vi "Main.vi"() -> ()   [LabVIEW 2020]
doc: "Ce VI modèle est conçu pour le modèle de conception Gestionnaire de messages dans une file d'attente.\n\nLa boucle de gestion d'événements génère des messages en fonction des actions sur l'interface utilisateur.\n\nLa boucle de gestion de messages traite les messages générés par la boucle de gestion d'événements ou par d'autres messages. Les messages sont des valeurs chaîne ; il est donc facile d'ajouter de nouveaux messages à la structure condition Conditions de messages de la boucle de gestion de messages Chaque cluster Message peut en outre fournir une valeur optionnelle pour Données de message, un variant qui peut être converti aux données requises pour un message spécifique."
uses:
  controls/Ctrl_RefPad.ctl
  controls/UI Data.ctl
  support/Message Queue/Enqueue Message (Single).vi
  <vilib>/Utility/error.llb/Error Cluster From Error Code.vi
  <vilib>/ErrorRing/Error Ring.xnode
  support/Message Queue/Message Queue.lvlib
  support/User Event - Stop/User Event - Stop.lvlib
panel:
  in  "Btn_Error_etat":bool caption="Error state"
  in  "Btn_Error":bool caption="Error"
  out "sortie d'erreur":errorcluster
  out "Display":cluster{"Num":dbl, "Char":string}
  in  "Pad":T1
  in  "Btn_Stop":bool
  # "Calculatrice"
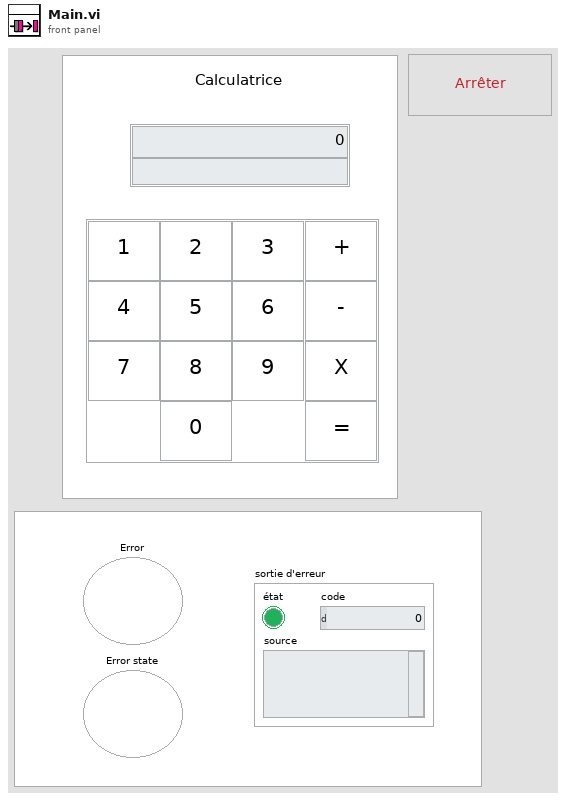
[diagram p1: front panel]
types:
  T1 = cluster{"Btn_1":bool, "Btn_2":bool, "Btn_3":bool, "Btn_4":bool, "Btn_5":bool, "Btn_6":bool, "Btn_7":bool, "Btn_8":bool, "Btn_9":bool, "Btn_0":bool, "Btn_+":bool, "Btn_-":bool, "Btn_X":bool, "Btn_=":bool}
  T2 = cluster{"état":bool, "code":i32, "source":string}
  T3 = typedef "Message Queue.lvlib/All Message Queues.ctl" = cluster{"IU":refnum<queue>}
  T4 = typedef "UI Data.ctl" = cluster{"Event":cluster{"Stop":refnum<user-event>}, "Data":cluster{"Display":cluster{"Num":dbl, "Char":string}, "memory":string}}
  T5 = typedef "Ctrl_RefPad.ctl" = cluster{"BTN_Ref":refnum<vi>, "CharPad":string}
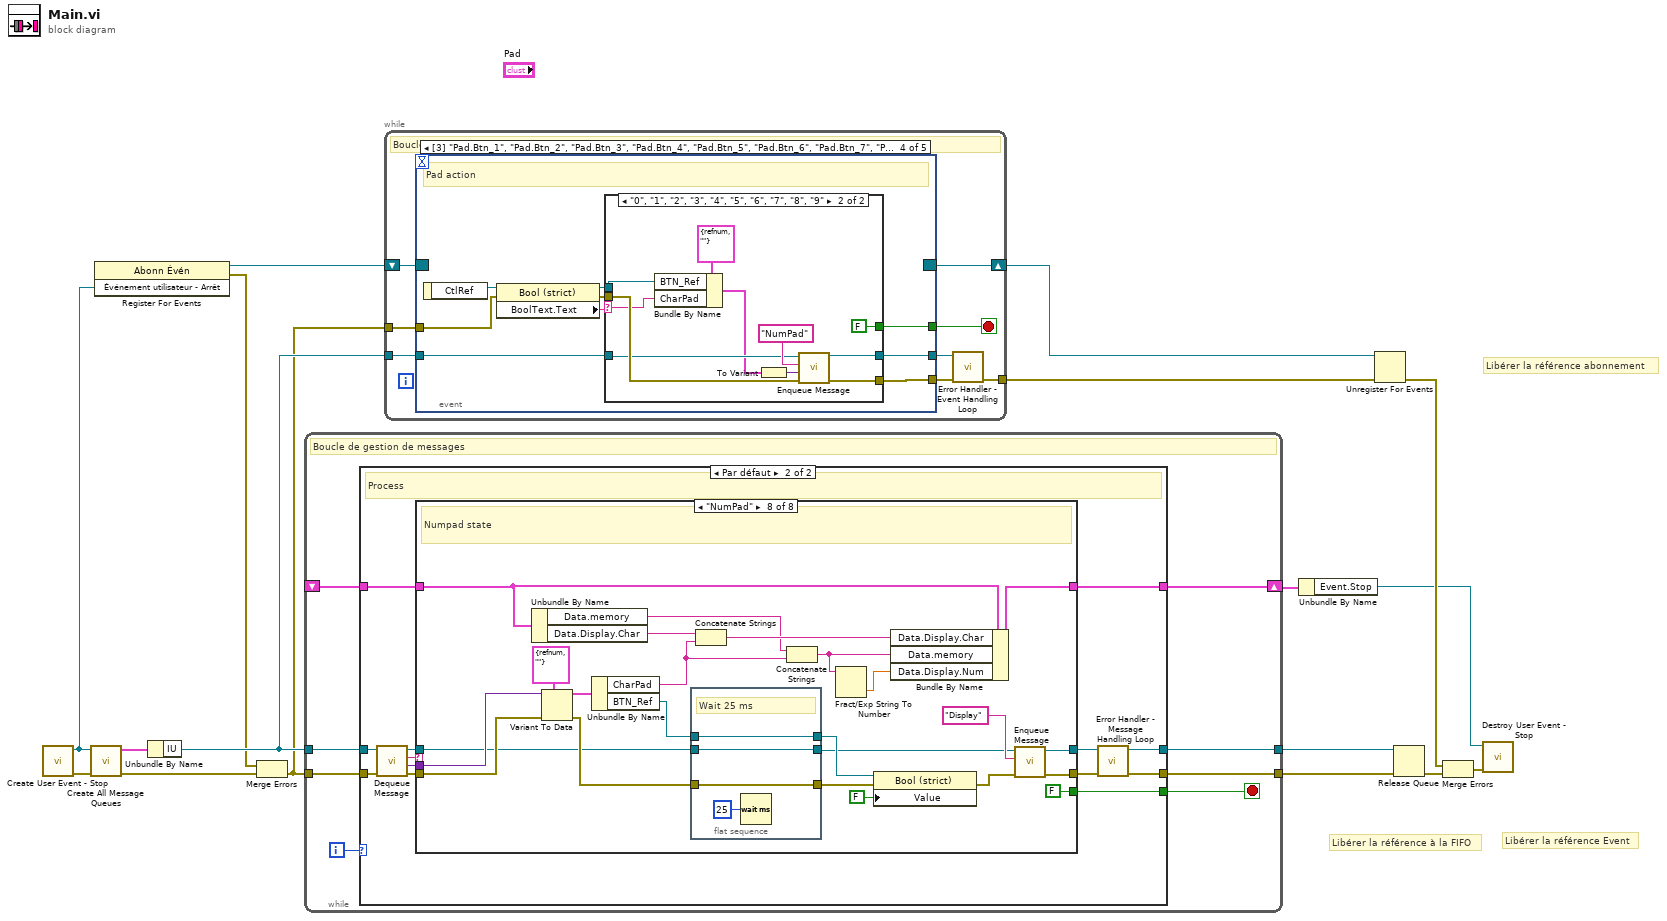
[diagram p0: block diagram]
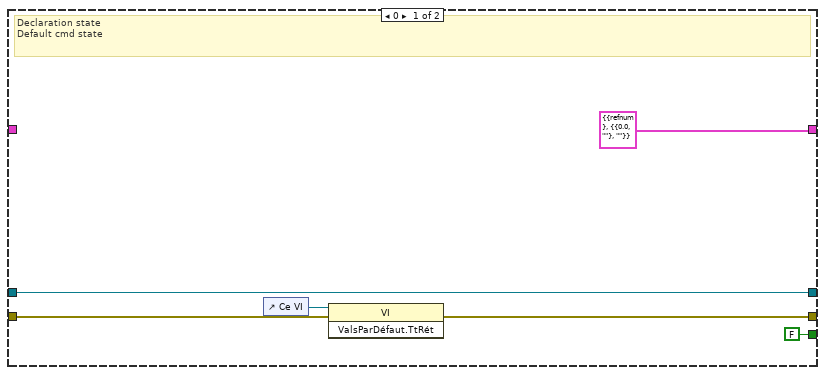
[diagram p2: hidden frame]
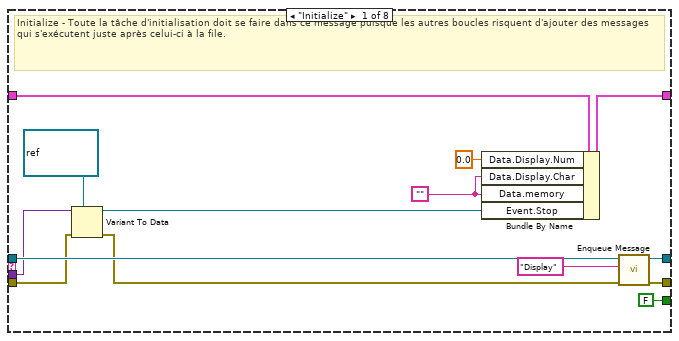
[diagram p3: hidden frame]
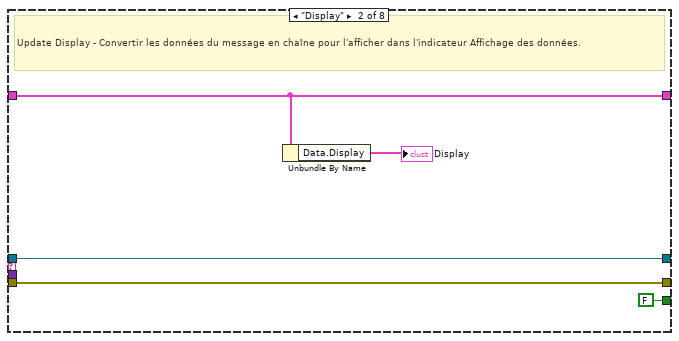
[diagram p4: hidden frame]
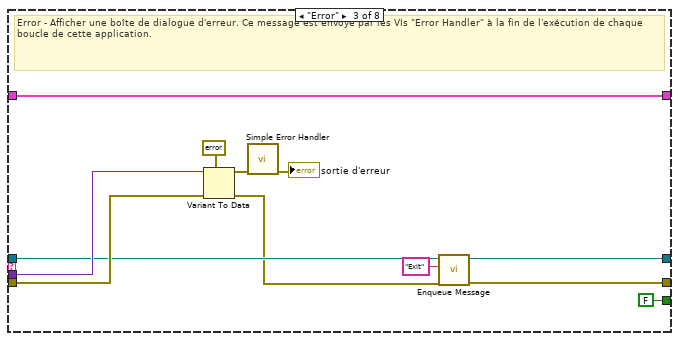
[diagram p5: hidden frame]
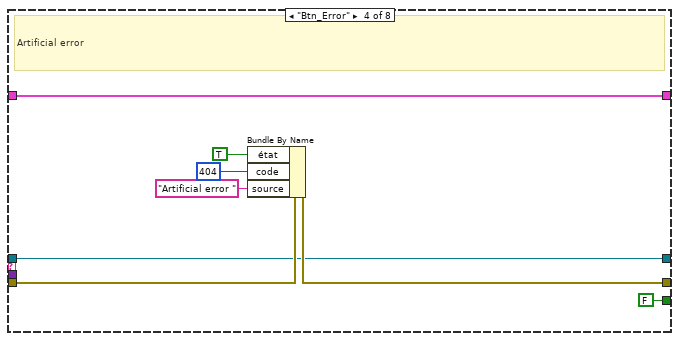
[diagram p6: hidden frame]
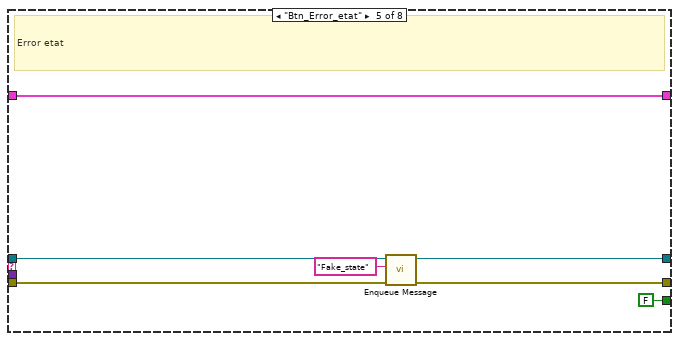
[diagram p7: hidden frame]
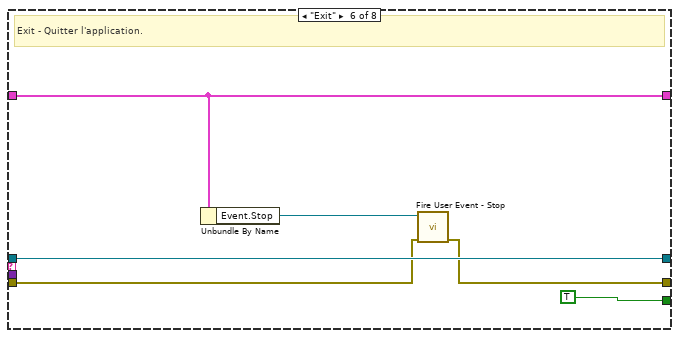
[diagram p8: hidden frame]
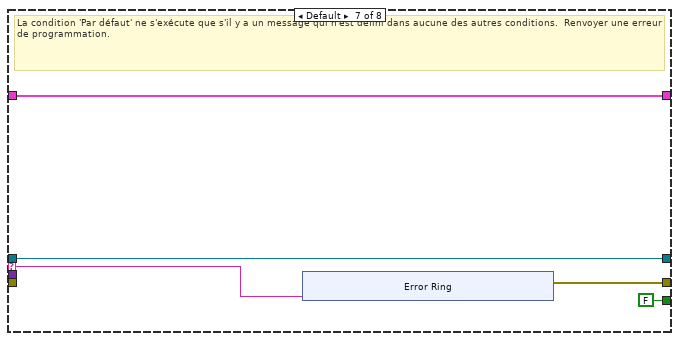
[diagram p9: hidden frame]
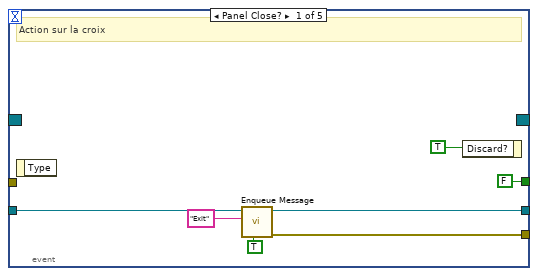
[diagram p10: hidden frame]
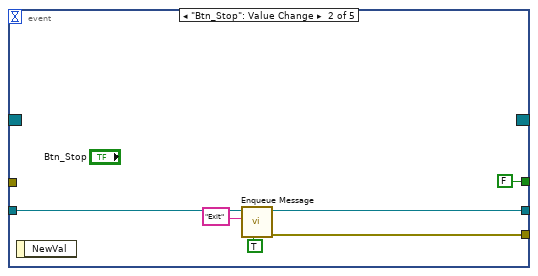
[diagram p11: hidden frame]
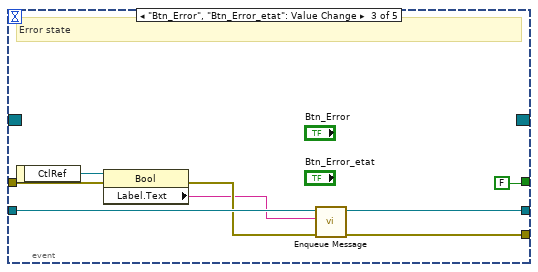
[diagram p12: hidden frame]
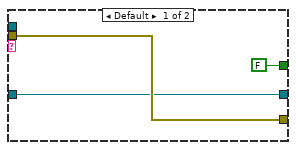
[diagram p13: hidden frame]
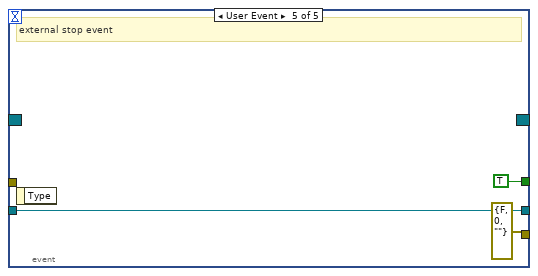
[diagram p14: hidden frame]
diagram:
  # "Libérer la référence abonnement"
  # "Libérer la référence Event"
  # "Libérer la référence à la FIFO"
  n1 = call "Create User Event - Stop.vi"() -> ("error out"=w14:T2, "Événement utilisateur - Arrêt"=w7:refnum<user-event>)  [unwired: 10 in]
  n2 = call "Create All Message Queues.vi"("error in (no error)"=w14, "Stop Event"=w7) -> ("error out"=w17:T2, "Fifo"=w16:T3)  [unwired: 8 in]
  n3 = register-events(w7) -> (reference out=w9:refnum<event-registration>, error out=w8:errorcluster)  [unwired: 2 in]
  n4 = Unbundle By Name(w16) -> ("IU"=w15:refnum<queue>)
  n5 = Merge Errors(w8, w17) -> (w1:errorcluster)
  n6 = while {
    tunnel: w15 -> [w21]
    shift-right: [w24] -> w6
    shift-left: _ -> [w25]
    tunnel: w1 -> [w22]
    tunnel: [w20] -> w3
    tunnel: [w19] -> w4
    i -> [w18]
    stop <- w23 stop-if-true
    # "Boucle de gestion de messages"
    n7 = case shown="Par défaut" w18 {
      tunnel: w25 -> [_ w44]
      tunnel: [T4 {"Event"={"Stop"=refnum}, "Data"={"Display"={"Num"=0.0, "Char"=""}, "memory"=""}} ("Data Cluster") w43] -> w24
      tunnel: [FALSE w42] -> w23
      tunnel: w22 -> [w27 w41]
      tunnel: w21 -> [w30 w37]
      tunnel: [w26 w35] -> w20
      tunnel: [w30 w32] -> w19
      frame 0 {
        # "Declaration state\nDefault cmd state"
        n8 = control-ref of="Ce VI"() -> (w28:refnum<vi>)
        n9 = invoke class="VI" method="ValsParDéfaut.TtRét"(reference=w28, error in=w27) -> (error out=w26:errorcluster)  [unwired: 1 in, 2 out]
      }
      frame Default {
        # "Process"
        n10 = call "Dequeue Message.vi"("error in (no error)"=w41, "File d'attente de messages"=w37) -> ("error out"=w40:T2, "Données de message"=w38:variant, "Message"=w39:string, "File d'attente de message dup."=w36:refnum<queue>)  [unwired: 6 in]
        n11 = case "Conditions des messages" shown="\"NumPad\"" w39 {
          selector: w39 -> [_ _ _ _ _ _ w99 _]
          tunnel: w36 -> [w54 w62 w69 w77 w86 w93 w97 w114]
          tunnel: w40 -> [w53 w61 w75 w83 w89 w92 _ w132]
          tunnel: [w58 w61 w66 w81 w88 w91 w100 w127] -> w34
          tunnel: w44 -> [w57 w60 w74 w82 w90 w95 w101 w126]
          tunnel: [w56 w60 w74 w82 w90 w95 w101 w125] -> w43
          tunnel: [FALSE FALSE FALSE FALSE FALSE TRUE FALSE FALSE] -> w42
          tunnel: w38 -> [w52 _ w73 _ _ _ _ w131]
          tunnel: [w47 w62 w68 w77 w87 w93 w97 w128] -> w33
          frame "Initialize" {
            w46 = ""
            # "Initialize - Toute la tâche d'initialisation doit se faire dans ce message puisque les autres boucles risquent d'ajouter des messages qui s'exécutent juste après celui-ci à la file."
            n12 = Variant To Data(error in=w53, type=refnum<user-event> refnum ("Stop Event"), Variant=w52) -> (data=w50:refnum<user-event>, error out=w49:errorcluster)
            n13 = Bundle By Name(cluster=w57, "Data.Display.Num"=0.0, "Data.Display.Char"=w46, "Data.memory"=w46, "Event.Stop"=w50) -> (w56:T4)
            n14 = call-poly "Enqueue Message.vi"("error in (no error)"=w49, "Message"="Display", "File d'attente de messages"=w54) -> ("error out"=w58:T2, "File d'attente de message dup."=w47:refnum<queue>)  [unwired: 7 in]
          }
          frame "Display" {
            # "Update Display - Convertir les données du message en chaîne pour l'afficher dans l'indicateur Affichage des données."
            n15 = Unbundle By Name(w60) -> ("Data.Display"=→"Display":cluster{"Num":dbl, "Char":string})
          }
          frame "Error" {
            # "Error - Afficher une boîte de dialogue d'erreur. Ce message est envoyé par les VIs \"Error Handler\" à la fin de l'exécution de chaque boucle de cette application."
            n16 = Variant To Data(error in=w75, type=errorcluster {"status"=FALSE, "code"=0, "source"=""} ("error constant"), Variant=w73) -> (data=w71:errorcluster, error out=w67:errorcluster)
            n17 = call <vilib>:"Simple Error Handler.vi"("error in (no error)"=w71) -> ("error out"=→"sortie d'erreur":errorcluster)  [unwired: 4 in, 4 out]
            n18 = call-poly "Enqueue Message.vi"("error in (no error)"=w67, "Message"="Exit", "File d'attente de messages"=w69) -> ("error out"=w66:T2, "File d'attente de message dup."=w68:refnum<queue>)  [unwired: 7 in]
          }
          frame "Btn_Error" {
            # "Artificial error"
            n19 = Bundle By Name(cluster=w83, "état"=TRUE, "code"=404, "source"="Artificial error ") -> (w81:T2)
          }
          frame "Btn_Error_etat" {
            # "Error etat"
            n20 = call-poly "Enqueue Message.vi"("error in (no error)"=w89, "Message"="Fake_state", "File d'attente de messages"=w86) -> ("error out"=w88:T2, "File d'attente de message dup."=w87:refnum<queue>)  [unwired: 7 in]
          }
          frame "Exit" {
            # "Exit - Quitter l'application."
            n21 = Unbundle By Name(w95) -> ("Event.Stop"=w94:refnum<user-event>)
            n22 = call "Fire User Event - Stop.vi"("error in (no error)"=w92, "Événement utilisateur - Arrêt"=w94) -> ("error out"=w91:T2)  [unwired: 9 in]
          }
          frame Default {
            # "La condition 'Par défaut' ne s'exécute que s'il y a un message qui n'est défini dans aucune des autres conditions.  Renvoyer une erreur de programmation."
            n23 = xnode ("Error Ring")("paramètre 0"=w99) -> ("sortie d'erreur"=w100:errorcluster)
          }
          frame "NumPad" {
            # "Numpad state"
            n24 = Unbundle By Name(w126) -> ("Data.memory"=w122:string, "Data.Display.Char"=w124:string)
            n25 = Variant To Data(error in=w132, type=T5 {"BTN_Ref"=refnum, "CharPad"=""} ("cluster"), Variant=w131) -> (data=w118:T5, error out=w115:errorcluster)
            n26 = Unbundle By Name(w118) -> ("CharPad"=w117:string, "BTN_Ref"=w116:refnum<vi>)
            n27 = flat-sequence {
              tunnel: w116 -> [w135]
              tunnel: [w135] -> w112
              tunnel: w115 -> [w134]
              tunnel: w114 -> [w133]
              tunnel: [w134] -> w113
              tunnel: [w133] -> w111
              frame #0 {
                # "Wait 25 ms"
                n28 = Wait (ms)(milliseconds to wait=u32 25 ("attente (ms)")) -> ()  [unwired: 1 out]
              }
            }
            n29 = Concatenate Strings(w124, w117) -> (w123:string)
            n30 = Concatenate Strings(w122, w117) -> (w121:string)
            n31 = Fract/Exp String To Number(string=w121) -> (number=w120:dbl)  [unwired: 3 in, 1 out]
            n32 = property class="Bool (strict)"(reference=w112, error in=w113, "Value"=FALSE ("Valeur")) -> (error out=w110:errorcluster)  [unwired: 1 out]
            n33 = Bundle By Name(cluster=w126, "Data.Display.Char"=w123, "Data.memory"=w121, "Data.Display.Num"=w120) -> (w125:T4)
            n34 = call-poly "Enqueue Message.vi"("error in (no error)"=w110, "Message"="Display", "File d'attente de messages"=w111) -> ("error out"=w127:T2, "File d'attente de message dup."=w128:refnum<queue>)  [unwired: 7 in]
          }
        }
        n35 = call "Error Handler - Message Handling Loop.vi"("error in (no error)"=w34, "File d'attente de messages"=w33) -> ("erreur en entrée dup."=w35:T2, "File d'attente de message dup."=w32:refnum<queue>)  [unwired: 8 in]
      }
    }
  }
  n36 = while {
    tunnel: w15 -> [w144]
    shift-right: [w142] -> w11
    shift-left: w9 -> [w143]
    tunnel: [w138] -> w10
    tunnel: w1 -> [w137]
    stop <- w140 stop-if-true
    # "Boucle de gestion d'événements"
    n37 = event shown="[3] \"Pad.Btn_1\", \"Pad.Btn_2\", \"Pad.Btn_3\", \"Pad.Btn_4\", \"Pad.Btn_5\", \"Pad.Btn_6\", \"Pad.Btn_7\", \"Pad.Btn_8\", \"Pad.Btn_9\", \"Pad.Btn_0\", \"Pad.Btn_+\": Valeur changée" {
      selector: w143 -> [_ _ _ _ _]
      dyn-events: [_ _ _ _ _] -> w142
      timeout: _ -> [_ _ _ _ _]
      tunnel: [FALSE ("Discard?") FALSE ("Discard?") FALSE w167 TRUE ("Discard?")] -> w140
      tunnel: w144 -> [w150 w157 w163 w169 w191]
      tunnel: [w149 w156 w158 w170 T2 {"état"=FALSE, "code"=0, "source"=""} ("error out")] -> w141
      tunnel: [w148 w155 w162 w168 w191] -> w139
      tunnel: w137 -> [_ _ w164 w173 _]
      event Panel Close? {
        # "Action sur la croix"
        n38 = event-data() -> ()  [unwired: 1 in, 1 out]
        n39 = call-poly "Enqueue Message.vi"("Message prioritaire ? (F)"=TRUE ("Priority Message? (F)"), "Message"="Exit", "File d'attente de messages"=w150) -> ("error out"=w149:T2, "File d'attente de message dup."=w148:refnum<queue>)  [unwired: 7 in]
        n40 = event-data ("Event Filter Node")("Discard?"=TRUE) -> ()  [unwired: 1 in, 1 out]
      }
      event "Btn_Stop": Value Change {
        n41 = event-data() -> ()  [unwired: 1 in, 1 out]
        n42 = call-poly "Enqueue Message.vi"("Message prioritaire ? (F)"=TRUE ("Priority Message? (F)"), "Message"="Exit", "File d'attente de messages"=w157) -> ("error out"=w156:T2, "File d'attente de message dup."=w155:refnum<queue>)  [unwired: 7 in]
      }
      event "Btn_Error", "Btn_Error_etat": Value Change {
        # "Error state"
        n43 = event-data() -> ("CtlRef"=w165:refnum<vi>)  [unwired: 1 in]
        n44 = property class="Bool"(reference=w165, error in=w164) -> (error out=w161:errorcluster, "Label.Text"=w160:string)  [unwired: 1 out]
        n45 = call-poly "Enqueue Message.vi"("error in (no error)"=w161, "Message"=w160, "File d'attente de messages"=w163) -> ("error out"=w158:T2, "File d'attente de message dup."=w162:refnum<queue>)  [unwired: 7 in]
      }
      event "Pad.Btn_1", "Pad.Btn_2", "Pad.Btn_3", "Pad.Btn_4", "Pad.Btn_5", "Pad.Btn_6", "Pad.Btn_7", "Pad.Btn_8", "Pad.Btn_9", "Pad.Btn_0", "Pad.Btn_+": Value Change {
        # "Pad action"
        n46 = event-data() -> ("CtlRef"=w174:refnum<vi>)  [unwired: 1 in]
        n47 = property class="Bool (strict)"(reference=w174, error in=w173) -> (reference out=w166:refnum<vi>, error out=w171:errorcluster, "BoolText.Text"=w172:string)
        n48 = case shown="\"0\", \"1\", \"2\", \"3\", \"4\", \"5\", \"6\", \"7\", \"8\", \"9\"" w172 {
          selector: w172 -> [_ w180]
          tunnel: w171 -> [w177 w187]
          tunnel: [w177 w186] -> w170
          tunnel: w169 -> [w176 w184]
          tunnel: [w176 w183] -> w168
          tunnel: [FALSE FALSE] -> w167
          tunnel: w166 -> [_ w181]
          frame Default {
          }
          frame "0", "1", "2", "3", "4", "5", "6", "7", "8", "9" {
            n49 = Bundle By Name(cluster=T5 {"BTN_Ref"=refnum, "CharPad"=""}, "BTN_Ref"=w181, "CharPad"=w180) -> (w179:T5)
            n50 = To Variant(anything=w179) -> (Variant=w185:variant)
            n51 = call-poly "Enqueue Message.vi"("error in (no error)"=w187, "Données de message"=w185, "Message"="NumPad", "File d'attente de messages"=w184) -> ("error out"=w186:T2, "File d'attente de message dup."=w183:refnum<queue>)  [unwired: 6 in]
          }
        }
      }
      event User Event {
        # "external stop event"
        n52 = event-data() -> ()  [unwired: 1 in, 1 out]
      }
    }
    n53 = call "Error Handler - Event Handling Loop.vi"("error in (no error)"=w141, "File d'attente de messages"=w139) -> ("erreur en entrée dup."=w138:T2)  [unwired: 8 in, 1 out]
  }
  n54 = Unbundle By Name(w6) -> ("Event.Stop"=w5:refnum<user-event>)
  n55 = Unregister For Events(event registration refnum=w11, error in=w10) -> (error out=w12:errorcluster)
  n56 = Release Queue(queue=w4, error in (no error)=w3) -> (error out=w2:errorcluster)  [unwired: 1 in, 2 out]
  n57 = Merge Errors(w12, w2) -> (w13:errorcluster)
  n58 = call "Destroy User Event - Stop.vi"("error in (no error)"=w13, "Événement utilisateur - Arrêt"=w5) -> ()  [unwired: 9 in, 1 out]
